vi "TestData_MySQL_InsertRecord.vi"(7 "TableName":string, 8 "error in (no error)":errorcluster, 9 "data_input":string, 10 "SQL File":path, 11 "Connection In":refnum<k7>) -> (0 "error out":errorcluster, 2 "ok?":bool, 3 "ADODB._Connection Out":refnum<k7>)   [LabVIEW 2012, in "Lib_UEL.ATE.lvlib" / "Lib_TestData.lvlib"]
uses:
  Lib_TestData.lvlib
panel:
  in  "ConnectionString":T1={"IP"="localhost", "Port"="3306", "DataBase"="uel_te", "User"="root", "Password"="alpha130723"}
  out "结果字符串":string
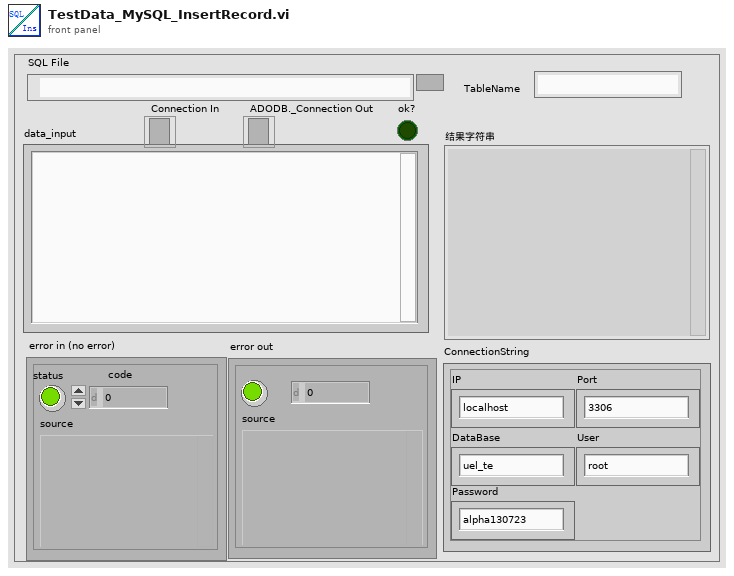
[diagram p1: front panel]
types:
  T1 = cluster{"IP":string, "Port":string, "DataBase":string, "User":string, "Password":string}
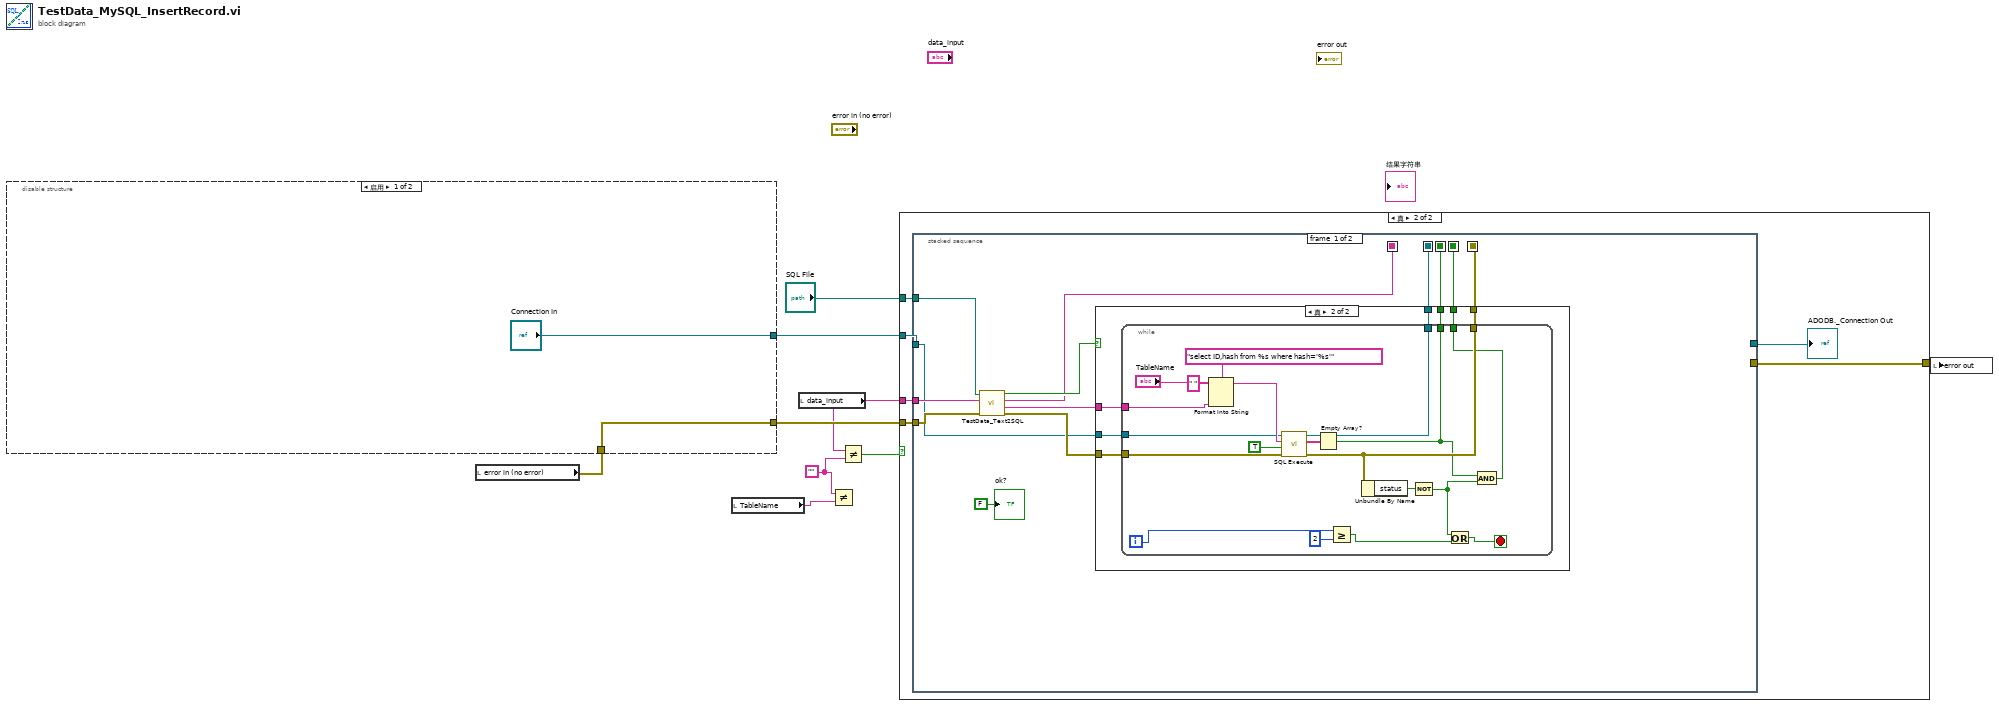
[diagram p0: block diagram]
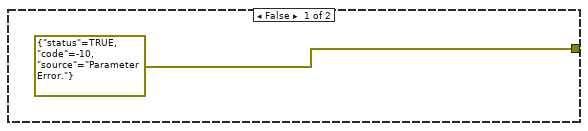
[diagram p2: hidden frame]
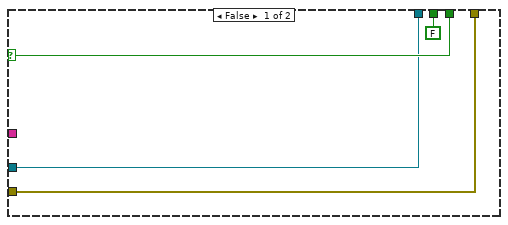
[diagram p3: hidden frame]
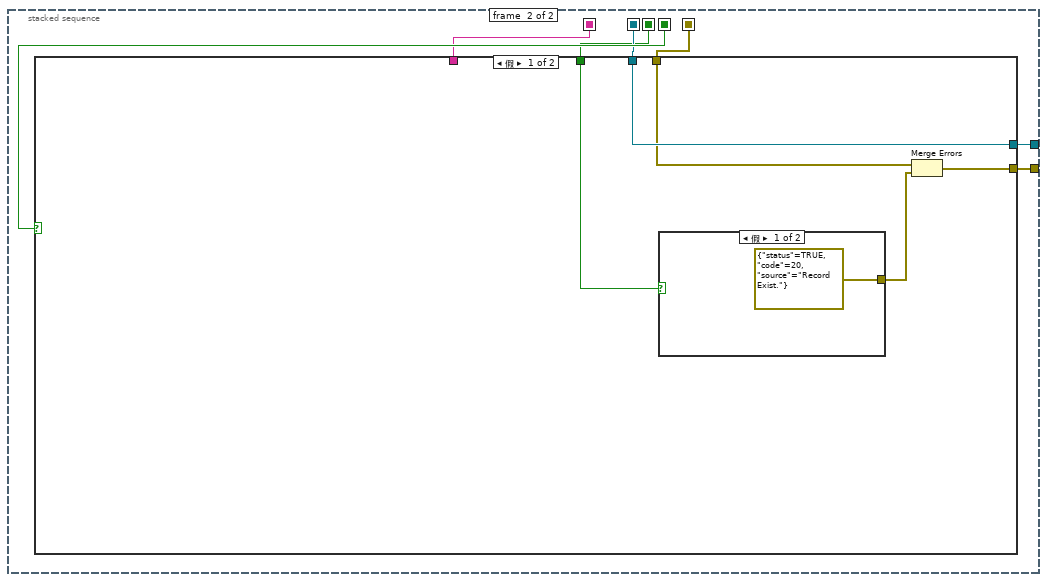
[diagram p4: hidden frame]
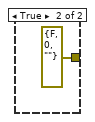
[diagram p5: hidden frame]
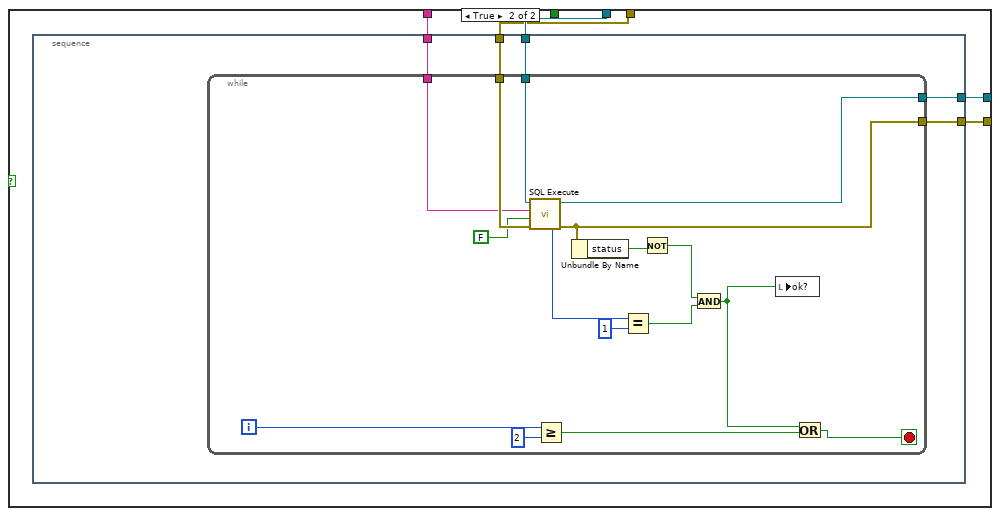
[diagram p6: hidden frame]
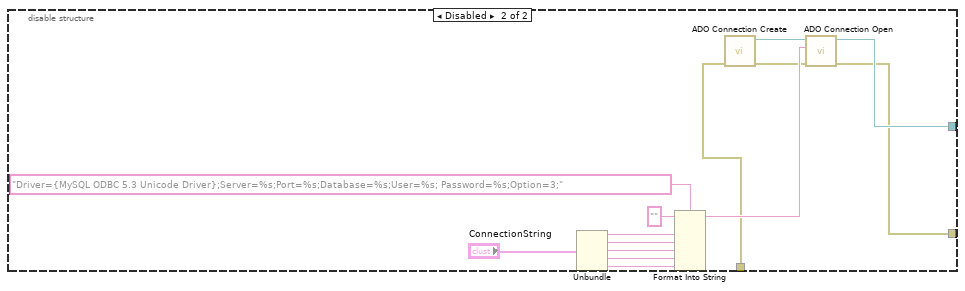
[diagram p7: hidden frame]
diagram:
  w2 = ""
  n1 = local read "error in (no error)"() -> (w6:errorcluster)
  n2 = disable-structure shown="启用" {
    disable-tunnel: ["Connection In" w14] -> w8
    disable-tunnel: w6 -> [w10 w13]
    disable-tunnel: [w10 w12] -> w5
    frame Enabled {
    }
    frame Disabled {
      n3 = Unbundle("ConnectionString") -> ("IP"=w18:string, "Port"=w19:string, "DataBase"=w20:string, "User"=w21:string, "Password"=w22:string)
      n4 = Format Into String(format string="Driver={MySQL ODBC 5.3 Unicode Driver};Server=%s;Port=%s;Database=%s;User=%s; Password=%s;Option=3;" ("格式字符串"), initial string="" ("初始字符串"), w18, w19, w20, w21, w22) -> (resulting string=w24:string)  [unwired: 1 in, 1 out]
      n5 = call <userlib>:"ADO Connection Create.vi"("error in (no error)"=w13) -> ("error out"=w23:errorcluster, "ADODB._Connection Out"=w25:refnum<k7>)  [unwired: 9 in]
      n6 = call <userlib>:"ADO Connection Open.vi"("error in (no error)"=w23, "ConnectionString"=w24, "ADODB._Connection In"=w25) -> ("error out"=w12:errorcluster, "ADODB._Connection Out"=w14:refnum<k7>)  [unwired: 7 in]
    }
  }
  n7 = local read "TableName"() -> (w4:string)
  n8 = local read "data_input"() -> (w3:string)
  n9 = Not Equal?(x=w2, y=w4) -> ()  [unwired: 1 out]
  n10 = Not Equal?(x=w3, y=w2) -> (x != y?=w1:bool)
  n11 = case shown="真" w1 {
    tunnel: [errorcluster {"status"=TRUE, "code"=-10, "source"="Parameter Error."} ("error out") w31] -> w9
    tunnel: w8 -> [_ w30]
    tunnel: "SQL File" -> [_ w29]
    tunnel: w5 -> [_ w28]
    tunnel: w3 -> [_ w27]
    frame False {
    }
    frame True {
      n12 = stacked-sequence {
        seq-local: [w45 _] -> [_ w82]
        seq-local: [w44 _] -> [_ w81]
        seq-local: [w43 _] -> [_ w80]
        seq-local: [w35 _] -> [_ w77]
        seq-local: [w33 _] -> [_ w76]
        tunnel: w28 -> [w41 _]
        tunnel: w30 -> [w36 _]
        tunnel: [_ w79] -> w32
        tunnel: [_ w78] -> w31
        tunnel: w27 -> [w40 _]
        tunnel: w29 -> [w42 _]
        frame #0 {
          n13 = call "TestData_Text2SQL.vi"("error in (no error)"=w41, "Record_Text"=w40, "SQL File"=w42) -> ("error out"=w39:errorcluster, "Hash_Code"=w38:string, "SQL Outpout"=w35:string, "ok?"=w37:bool)  [unwired: 5 in]
          n14 = case shown="真" w37 {
            selector: w37 -> [w49 _]
            tunnel: [w49 w56] -> w45
            tunnel: [w48 w55] -> w44
            tunnel: [w47 w54] -> w43
            tunnel: w39 -> [w47 w53]
            tunnel: w38 -> [_ w52]
            tunnel: w36 -> [w48 w51]
            tunnel: [FALSE ("empty?") w50] -> w33
            frame False {
            }
            frame True {
              n15 = while {
                tunnel: [w60] -> w56
                tunnel: [w71] -> w55
                tunnel: [w63] -> w54
                tunnel: w53 -> [w70]
                tunnel: w52 -> [w58]
                tunnel: w51 -> [w69]
                tunnel: [w59] -> w50
                i -> [w67]
                stop <- w64 stop-if-true
                n16 = Format Into String(format string="select ID,hash from %s where hash='%s'" ("格式字符串"), initial string=" " ("字符串"), "TableName", w58) -> (resulting string=w73:string)  [unwired: 1 in, 1 out]
                n17 = call <userlib>:"SQL Execute.vi"("error in (no error)"=w70, "Return Data (T)"=TRUE, "Command Text"=w73, "ADODB._Connection In"=w69) -> ("error out"=w63:errorcluster, "Data"=w68:string[][], "ADODB._Connection Out"=w71:refnum<k7>)  [unwired: 4 in, 1 out]
                n18 = Empty Array?(array=w68) -> (empty?=w59:bool)
                n19 = Greater Or Equal?(x=w67, y=2) -> (x >= y?=w65:bool)
                n20 = Unbundle By Name(w63) -> ("status"=w62:bool)
                n21 = Not(x=w62) -> (.not. x?=w61:bool)
                n22 = Or(x=w61, y=w65) -> (x .or. y?=w64:bool)
                n23 = And(x=w59, y=w61) -> (x .and. y?=w60:bool)
              }
            }
          }
          "ok?" <- FALSE ("ok?")
        }
        frame #1 {
          n24 = case shown="假" w82 {
            tunnel: w81 -> [w87 w94]
            tunnel: w80 -> [w85 w93]
            tunnel: [w87 w92] -> w79
            tunnel: [w84 w91] -> w78
            tunnel: w77 -> [_ w90]
            tunnel: w76 -> [w83 _]
            frame False {
              n25 = case shown="假" w83 {
                tunnel: [errorcluster {"status"=TRUE, "code"=20, "source"="Record Exist."} ("error out") errorcluster {"status"=FALSE, "code"=0, "source"=""} ("error out")] -> w86
                frame False {
                }
                frame True {
                }
              }
              n26 = Merge Errors(w85, w86) -> (w84:errorcluster)
            }
            frame True {
              n27 = stacked-sequence {
                tunnel: w94 -> [w99]
                tunnel: w93 -> [w98]
                tunnel: [w96] -> w92
                tunnel: [w95] -> w91
                tunnel: w90 -> [w97]
                frame #0 {
                  n28 = while {
                    tunnel: w99 -> [w115]
                    tunnel: w98 -> [w114]
                    tunnel: w97 -> [w112]
                    tunnel: [w111] -> w96
                    tunnel: [w104] -> w95
                    i -> [w108]
                    stop <- w105 stop-if-true
                    n29 = call <userlib>:"SQL Execute.vi"("error in (no error)"=w114, "Return Data (T)"=FALSE, "Command Text"=w112, "ADODB._Connection In"=w115) -> ("error out"=w104:errorcluster, "Rows Affected"=w110:i32, "ADODB._Connection Out"=w111:refnum<k7>)  [unwired: 4 in, 1 out]
                    n30 = Greater Or Equal?(x=w108, y=2) -> (x >= y?=w106:bool)
                    n31 = Unbundle By Name(w104) -> ("status"=w103:bool)
                    n32 = Equal?(x=w110, y=1) -> (x = y?=w101:bool)
                    n33 = Not(x=w103) -> (.not. x?=w102:bool)
                    n34 = And(x=w102, y=w101) -> (x .and. y?=w100:bool)
                    n35 = local write "ok?"(w100) -> ()
                    n36 = Or(x=w100, y=w106) -> (x .or. y?=w105:bool)
                  }
                }
              }
            }
          }
        }
      }
      "ADODB._Connection Out" <- w32
    }
  }
  n37 = local write "error out"(w9) -> ()
